vi "Main Page.vi"(8 "error in (no error)":errorcluster, 11 "Node Ptr":T1 format="%.0x") -> (0 "error out":errorcluster)   [LabVIEW 2021, in "NI 272x Resistive Simulation Custom Device Configuration.lvlib"]
uses:
  NI 272x Resistive Simulation Custom Device Configuration.lvlib
  Program Files/National Instruments/LabVIEW 2021/vi.lib/NI VeriStand/Custom Device API/Custom Device Item Ref.ctl
  Globals/Names.vi
  Program Files/National Instruments/LabVIEW 2021/vi.lib/NI VeriStand/Custom Device API/Get Item Property (Double).vi
  Program Files/National Instruments/LabVIEW 2021/vi.lib/NI VeriStand/Custom Device API/Get Item Property (String).vi
  Program Files/National Instruments/LabVIEW 2021/vi.lib/NI VeriStand/Custom Device API/Set Item Property (String).vi
  Program Files/National Instruments/LabVIEW 2021/vi.lib/NI VeriStand/Custom Device API/Set Item Property (Double).vi
  Program Files/National Instruments/LabVIEW 2021/vi.lib/NI VeriStand/Custom Device API/Custom Device API.lvlib
  NI 272x Resistive Simulation Custom Device Shared.lvlib
panel:
  in  "Update rate (Hz)":dbl=1.0 min=1.0 max=1000.0
  in  "272x Device Name":string
  in  "Header":cluster{"Section Name":string}={"Section Name"="Resistive Simulation Custom Device Settings"}
  in  "Description":string
  in  "Name":string
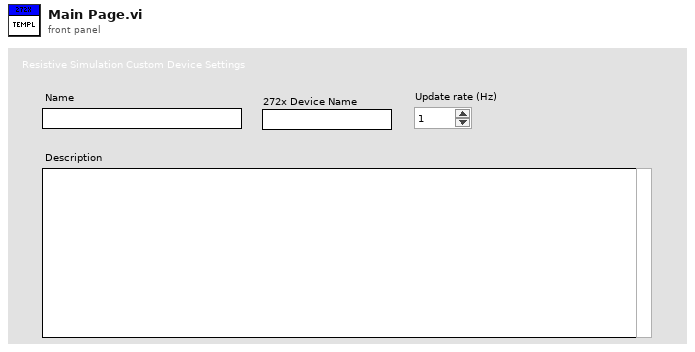
[diagram p1: front panel]
types:
  T1 = typedef "Custom Device API.lvlib/Custom Device Item Ref.ctl" = u64
  T2 = typedef "Custom Device API.lvlib/Custom Device Item Info.ctl" = cluster{"Name":string, "Is Channel":bool, "GUID":string, "Is Waveform":bool}
  T3 = typedef "Custom Device API.lvlib/Custom Device Commands.ctl" = enum16{"Default", "Item renamed", "Shutdown", "Dynamic button pressed"}
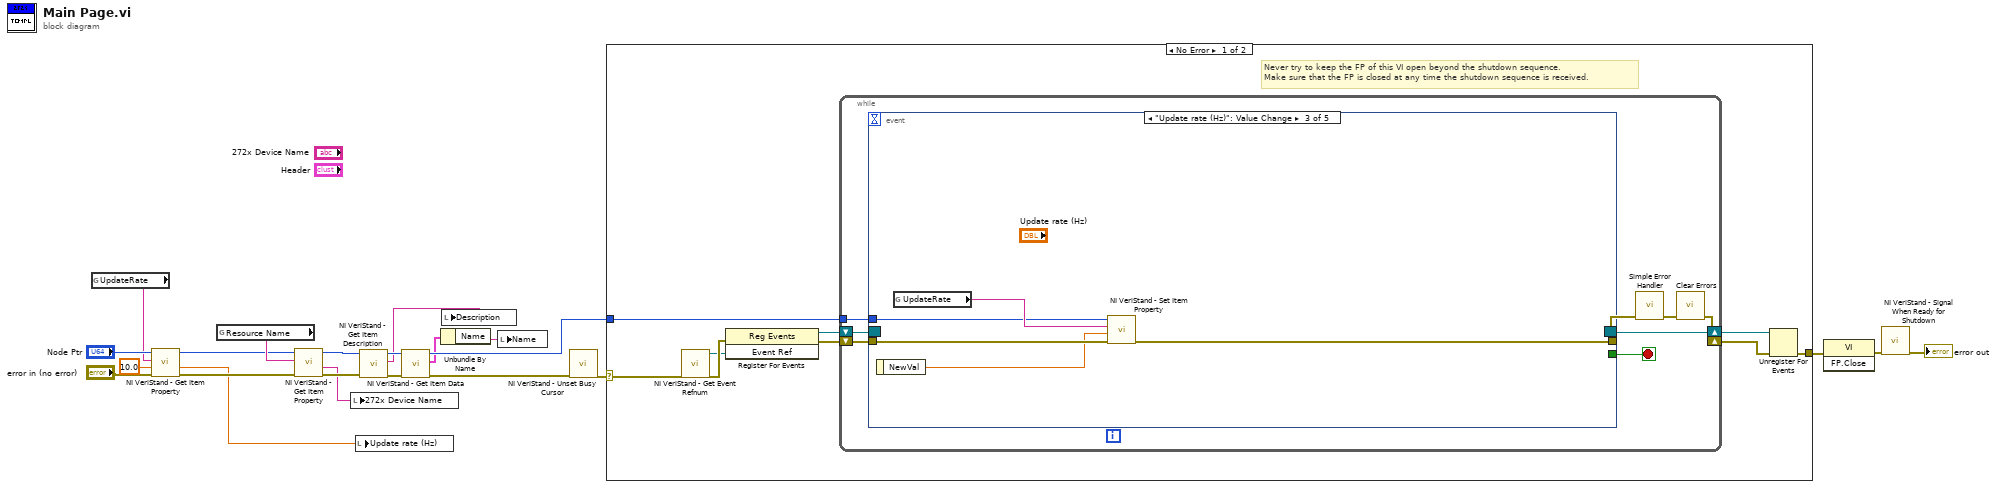
[diagram p0: block diagram]
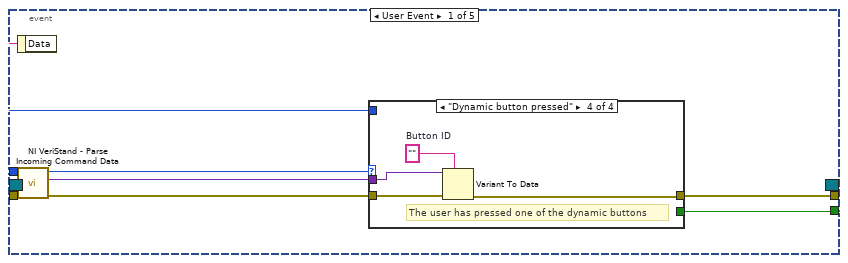
[diagram p2: hidden frame]
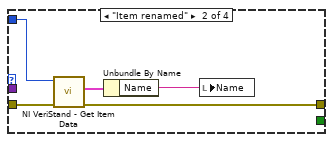
[diagram p4: hidden frame]
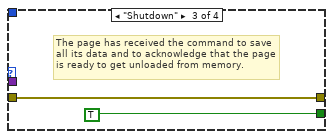
[diagram p5: hidden frame]
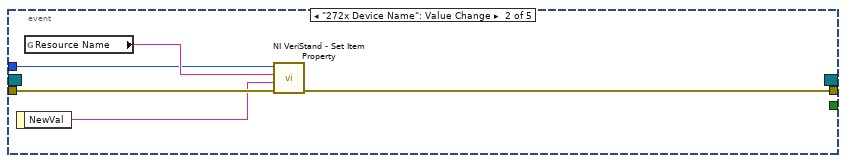
[diagram p6: hidden frame]
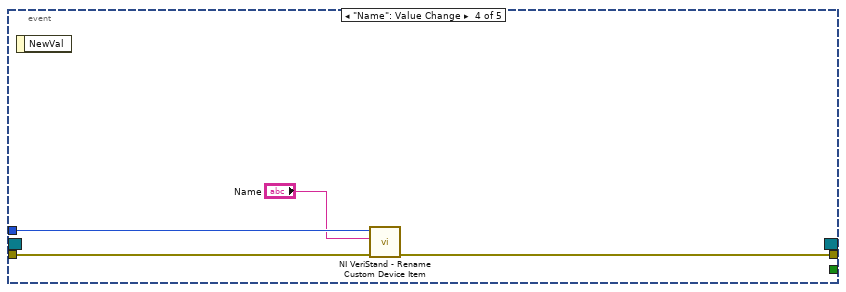
[diagram p7: hidden frame]
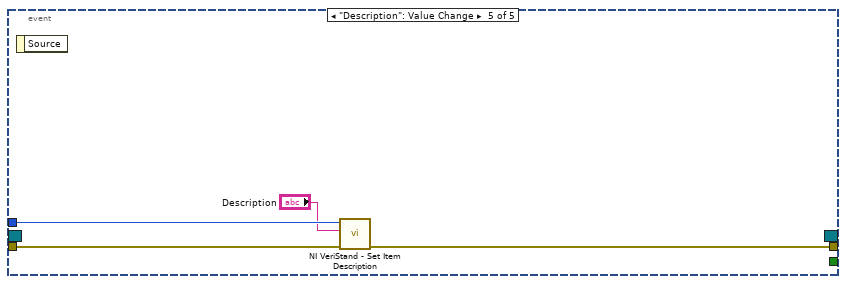
[diagram p8: hidden frame]
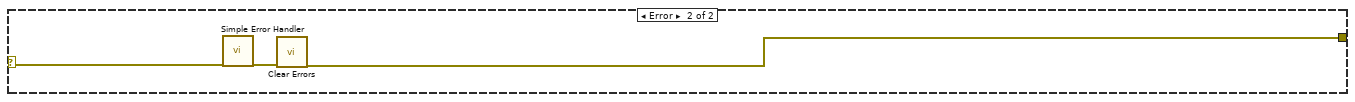
[diagram p9: hidden frame]
diagram:
  n1 = global read "Names.vi" "UpdateRate"() -> (w3:string)
  n2 = call-poly "NI VeriStand - Get Item Property.vi"("error in (no error)"="error in (no error)", "Default Value"=10.0, "Property Name"=w3, "Item Ref in"="Node Ptr") -> ("error out"=w6:errorcluster, "Value"=w1:dbl, "Item Ref out"=w4:T1)  [unwired: 4 in, 1 out]
  n3 = global read "Names.vi" "Resource Name"() -> (w10:string)
  n4 = call-poly "NI VeriStand - Get Item Property.vi"("error in (no error)"=w6, "Property Name"=w10, "Item Ref in"=w4) -> ("error out"=w8:errorcluster, "Value"=w7:string, "Item Ref out"=w9:T1)  [unwired: 5 in, 1 out]
  n5 = local write "272x Device Name"(w7) -> ()
  n6 = local write "Update rate (Hz)"(w1) -> ()
  n7 = call "NI VeriStand - Get Item Description.vi"("error in (no error)"=w8, "Item Ref in"=w9) -> ("error out"=w13:errorcluster, "Description"=w14:string, "Item Ref out"=w15:T1)  [unwired: 7 out]
  n8 = call "NI VeriStand - Get Item Data.vi"("error in (no error)"=w13, "Item Ref in"=w15) -> ("error out"=w16:errorcluster, "Item Info"=w12:T2, "Item Ref out"=w17:T1)  [unwired: 7 out]
  n9 = Unbundle By Name(w12) -> ("Name"=w11:string)
  n10 = local write "Description"(w14) -> ()
  n11 = local write "Name"(w11) -> ()
  n12 = call "NI VeriStand - Unset Busy Cursor.vi"("error in (no error)"=w16) -> ("error out"=w19:errorcluster)  [unwired: 10 out]
  n13 = case shown="No Error" w19 {
    selector: w19 -> [w23 w80]
    tunnel: [w28 w78] -> w22
    tunnel: w17 -> [w24 _]
    frame No Error {
      # "Never try to keep the FP of this VI open beyond the shutdown sequence.\nMake sure that the FP is closed at any time the shutdown sequence is received."
      n14 = call "NI VeriStand - Get Event Refnum.vi"("error in (no error)"=w23) -> ("error out"=w31:errorcluster, "Event Ref"=w27:refnum<user-event>)  [unwired: 9 out]
      n15 = register-events(error in=w31, w27) -> (reference out=w25:refnum<event-registration>, error out=w26:errorcluster)  [unwired: 1 in]
      n16 = while {
        tunnel: w24 -> [w36]
        shift-right: [w32] -> w29
        shift-left: w26 -> [w33]
        shift-right: [w39] -> w30
        shift-left: w25 -> [w38]
        stop <- w37 stop-if-true
        n17 = event shown="[2] \"Update rate (Hz)\": Value Change" {
          selector: w38 -> [_ _ _ _ _]
          dyn-events: [_ _ _ _ _] -> w39
          timeout: _ -> [_ _ _ _ _]
          tunnel: w33 -> [w47 w62 w67 w73 w76]
          tunnel: [w43 _ _ _ _] -> w37
          tunnel: [w42 w61 w66 w72 w75] -> w34
          tunnel: w36 -> [w41 w63 w68 w71 w77]
          event User Event {
            n18 = event-data() -> ("Data"=w46:string)  [unwired: 1 out]
            n19 = call "NI VeriStand - Parse Incoming Command Data.vi"("error in (no error)"=w47, "Incoming data"=w46) -> ("error out"=w45:errorcluster, "Outgoing data"=w40:variant, "Action"=w44:T3)  [unwired: 7 out]
            n20 = case shown="\"Dynamic button pressed\"" w44 {
              tunnel: w45 -> [w48 w53 w54 w59]
              tunnel: [_ _ TRUE _] -> w43
              tunnel: [w48 w50 w54 w56] -> w42
              tunnel: w41 -> [_ w52 _ _]
              tunnel: w40 -> [_ _ _ w58]
              frame "Default", Default {
              }
              frame "Item renamed" {
                n21 = call "NI VeriStand - Get Item Data.vi"("error in (no error)"=w53, "Item Ref in"=w52) -> ("error out"=w50:errorcluster, "Item Info"=w51:T2)  [unwired: 8 out]
                n22 = Unbundle By Name(w51) -> ("Name"=w49:string)
                n23 = local write "Name"(w49) -> ()
              }
              frame "Shutdown" {
                # "The page has received the command to save all its data and to acknowledge that the page is ready to get unloaded from memory."
              }
              frame "Dynamic button pressed" {
                w57 = ""  # Button ID
                # "The user has pressed one of the dynamic buttons"
                n24 = Variant To Data(error in=w59, type=w57, Variant=w58) -> (error out=w56:errorcluster)  [unwired: 1 out]
              }
            }
          }
          event "272x Device Name": Value Change {
            n25 = event-data() -> ("NewVal"=w60:string)  [unwired: 1 out]
            n26 = global read "Names.vi" "Resource Name"() -> (w64:string)
            n27 = call-poly "NI VeriStand - Set Item Property.vi"("error in (no error)"=w62, "Value"=w60, "Property Name"=w64, "Item Ref in"=w63) -> ("error out"=w61:errorcluster)  [unwired: 5 in, 2 out]
          }
          event "Update rate (Hz)": Value Change {
            n28 = event-data() -> ("NewVal"=w65:dbl)  [unwired: 1 out]
            n29 = global read "Names.vi" "UpdateRate"() -> (w69:string)
            n30 = call-poly "NI VeriStand - Set Item Property.vi"("error in (no error)"=w67, "Value"=w65, "Property Name"=w69, "Item Ref in"=w68) -> ("error out"=w66:errorcluster)  [unwired: 5 in, 2 out]
          }
          event "Name": Value Change {
            n31 = event-data() -> ()  [unwired: 2 out]
            n32 = call "NI VeriStand - Rename Custom Device Item.vi"("error in (no error)"=w73, "New Name"="Name", "Item Ref in"=w71) -> ("error out"=w72:errorcluster)  [unwired: 1 in, 7 out]
          }
          event "Description": Value Change {
            n33 = event-data() -> ()  [unwired: 2 out]
            n34 = call "NI VeriStand - Set Item Description.vi"("error in (no error)"=w76, "Description"="Description", "Item Ref in"=w77) -> ("error out"=w75:errorcluster)  [unwired: 8 out]
          }
        }
        n35 = call <vilib>:"Simple Error Handler.vi"("error in (no error)"=w34) -> ("error out"=w35:errorcluster)  [unwired: 1 in, 7 out]
        n36 = call <vilib>:"Clear Errors.vi"("error in (no error)"=w35) -> ("error out"=w32:errorcluster)  [unwired: 1 in, 5 out]
      }
      n37 = Unregister For Events(event registration refnum=w30, error in=w29) -> (error out=w28:errorcluster)
    }
    frame Error {
      n38 = call <vilib>:"Simple Error Handler.vi"("error in (no error)"=w80) -> ("error out"=w79:errorcluster)  [unwired: 1 in, 7 out]
      n39 = call <vilib>:"Clear Errors.vi"("error in (no error)"=w79) -> ("error out"=w78:errorcluster)  [unwired: 1 in, 5 out]
    }
  }
  n40 = invoke class="VI" method="FP.Close"(error in=w22) -> (error out=w21:errorcluster)  [unwired: 2 in, 2 out]
  n41 = call "NI VeriStand - Signal When Ready for Shutdown.vi"("error in (no error)"=w21) -> ("error out"=→"error out":errorcluster)  [unwired: 10 out]
